vi "swerve-drive-pose-est-test.vi"(8 "error in (no error)":errorcluster) -> (0 "error out":errorcluster, 3 "Test Passed":bool)   [LabVIEW 2019]
uses:
  <vilib>/Rock Robotics/WPI/ThirdParty/JAS_Junk/TrajLib/MatBuilder_Create.vi
  <vilib>/Rock Robotics/WPI/ThirdParty/JAS_Junk/TrajLib/MatrixHelper_CoerceSize.vi
  <vilib>/Rock Robotics/WPI/ThirdParty/JAS_Junk/TrajLib/Util_CalcDist.vi
  <vilib>/Analysis/1siggen.llb/Gaussian White Noise.vi
  <vilib>/Rock Robotics/WPI/ThirdParty/JAS_Junk/TrajLib/Trajectory_Library.lvlib
panel:
  out "BenchProcessing Timer Per Pass":dbl
  out "BenchTotalTime":dbl
  out "BenchTotalPasses":dbl
  out "MaxErrPassed":bool
  out "TotalPassed":bool
  out "EerrSumNormalized":dbl
  out "Error Sum":dbl
  out "Max Error":dbl
  out "Using Vision":bool
  in  "UseVIsion":bool=TRUE
  out "VIsionUpdates":i32
  out "TotalTImeSecs":dbl
  out "Position Graph":cluster{dbl[], dbl[]}[](graph)
  out "PoesEstCreateErr":bool
  # "< 0.42"
  # "< 0.25"
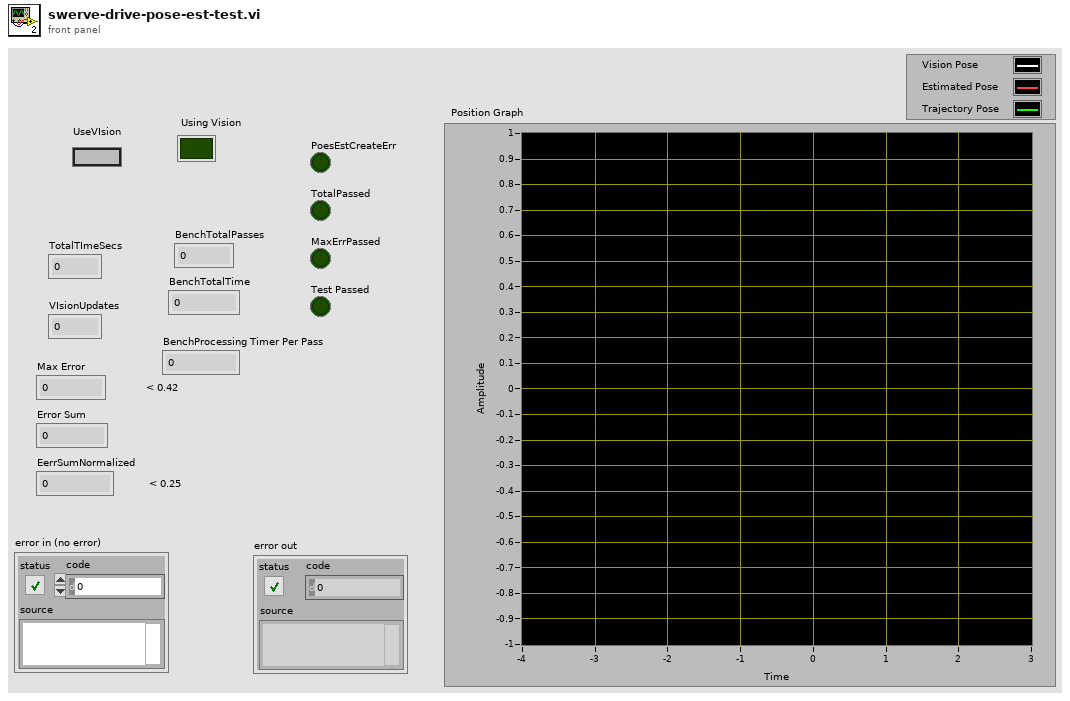
[diagram p1: front panel]
types:
  T1 = typedef "Trajectory_Library.lvlib/TRANSLATION2D.ctl" = cluster{"X":dbl, "Y":dbl}
  T2 = typedef "Trajectory_Library.lvlib/ROTATION2D.ctl" = cluster{"VALUE":dbl, "COS":dbl, "SIN":dbl}
  T3 = typedef "Trajectory_Library.lvlib/POSE2D.ctl" = cluster{"TRANSLATION":T1, "ROTATION":T2}
  T4 = typedef "NI_Matrix.lvlib/RealMatrix.ctl" = dbl[][]
  T5 = typedef "Trajectory_Library.lvlib/SWERVE_DRIVE_KINEMATICS.ctl" = cluster{"NumModules":i32, "InverseKinematics":T4, "ForwardKinematics":T4, "Modules":T1[], "PrevCoR":T1}
  T6 = typedef "Trajectory_Library.lvlib/TRAJ_CONFIG.ctl" = cluster{"MaxVelocity":dbl, "Max Acceleration":dbl, "StartVelocity":dbl, "End Velocity":dbl, "Reversed":bool, "DiffDrKineConstntDefined":bool, "CentAcellConstntDefined":bool, "DiffDrVoltConstntDefined":bool, "DIFF_DRIVE_KINE_CONSTRAINT":T7, "CENTRIPETAL_ACCEL_CONSTRAINT":T9, "SwerveDrKineConstntDefined":bool, "SWERVE_DRIVE_KINE_CONSTRAINT":T10, "DIFF_DRIVE_VOLTAGE_CONSTRAINT":T11, "MECANUM_DRIVE_KINE_CONSTRAINT":T13, "MecanumDrKineConstntDefined":bool}
  T7 = typedef "Trajectory_Library.lvlib/TRAJ_CONSTRAINT_DIIF_DRIVE_KINEMATICS.ctl" = cluster{"Max Speed (M/S)":dbl, "DIFF_DRIVE_KINEMATICS":T8, "Max Accel (M/S2)":dbl}
  T8 = typedef "Trajectory_Library.lvlib/DIFF_DRIVE_KINEMATICS.ctl" = cluster{"TrackWidth_Meters":dbl}
  T9 = typedef "Trajectory_Library.lvlib/TRAJ_CONSTRAINT_CENTRIPETAL_ACCEL.ctl" = cluster{"Max Cent Accel":dbl}
  T10 = typedef "Trajectory_Library.lvlib/TRAJ_CONSTRAINT_SWERVE_DRIVE_KINEMATICS.ctl" = cluster{"Max Speed (M/S)":dbl, "SwerveKinematics":T5}
  T11 = typedef "Trajectory_Library.lvlib/TRAJ_CONSTRAINT_DIIF_DRIVE_VOLTAGE.ctl" = cluster{"Max Voltage":dbl, "DIFF_DRIVE_KINEMATICS":T8, "SIMPLE_MOTOR_FF":T12}
  T12 = typedef "Trajectory_Library.lvlib/SIMPLE_MOTOR_FF.ctl" = cluster{"Ks":dbl, "Kv":dbl, "Ka":dbl}
  T13 = typedef "Trajectory_Library.lvlib/TRAJ_CONSTRAINT_MECA_DRIVE_KINEMATICS.ctl" = cluster{"Max Speed (M/S)":dbl, "MECA_DRIVE_KINEMATICS":T14}
  T14 = typedef "Trajectory_Library.lvlib/MECA_DRIVE_KINEMATICS.ctl" = cluster{"FrontLeft":T1, "FrontRight":T1, "RearLeft":T1, "RearRight":T1, "InverseKinematics":T4, "ForwardKinematics":T4, "PrevCoR":T1}
  T15 = typedef "Trajectory_Library.lvlib/SWERVE_DRIVE_POSE_EST.ctl" = cluster{"M_VisionContR":T4, "m_nominal_dT":dbl, "m_PrevTime_Sec":dbl, "m_GyroOffset":T2, "m_PrevAngle":T2, "m_Observer":T16, "m_latencyCompensator":T19, "m_kinematics":T5}
  T16 = typedef "Trajectory_Library.lvlib/UNSCENTED_KALMAN_FILTER.ctl" = cluster{"m_P":T4, "m_xHat":T4, "States":i32, "Outputs":i32, "m_ContR":T4, "m_ContQ":T4, "m_SigmasF":T4, "m_dT_Sec":dbl, "MERWE_SCALED_SIGMA_PTS":T17, "meanFuncX":T18, "meanFuncY":T18, "residualFuncX":T18, "residualFuncY":T18, "addFuncX":T18, "addFuncXExtra":variant, "residualFuncYExtra":variant, "residualFuncXExtra":variant, "MeanFuncYExtra":variant, "MeanFuncXExtra":variant, "Inputs":i32}
  T17 = typedef "Trajectory_Library.lvlib/MERWE_SCALED_SIGMA_PTS.ctl" = cluster{"m_Wm":T4, "States":i32, "Alpha":dbl, "m_Wc":T4, "Kappa":i32}
  T18 = typedef "Trajectory_Library.lvlib/CALLBACK_FUNC_TYPE.ctl" = refnum<vi>
  T19 = typedef "Trajectory_Library.lvlib/KALMAN_FILTER_LATENCY_COMP.ctl" = cluster{"m_pastObserverSnapshots ":T20[]}
  T20 = typedef "Trajectory_Library.lvlib/OBSERVER_SNAP_LIST_ITEM.ctl" = cluster{"TimeStamp":dbl, "OBSERVER_SNAPSHOT":T21}
  T21 = typedef "Trajectory_Library.lvlib/OBSERVER_SNAPSHOT.ctl" = cluster{"ErrorCoVariance":T4, "xHat":T4, "LocalMeasurements":T4, "Inputs":T4}
  T22 = typedef "Trajectory_Library.lvlib/TRAJECTORY.ctl" = cluster{"TotalTImeSecs":dbl, "States":T23[]}
  T23 = typedef "Trajectory_Library.lvlib/TRAJ_STATE.ctl" = cluster{"TimeSeconds":dbl, "Velocity":dbl, "Acceleration":dbl, "POSE":T3, "Curvature":dbl}
  T24 = typedef "Trajectory_Library.lvlib/CHASSIS_SPEEDS.ctl" = cluster{"vX":dbl, "vY":dbl, "vOmega":dbl}
  T25 = typedef "Trajectory_Library.lvlib/SWERVE_DRIVE_MODULE_STATE.ctl" = cluster{"Speed":dbl, "Angle":T2}
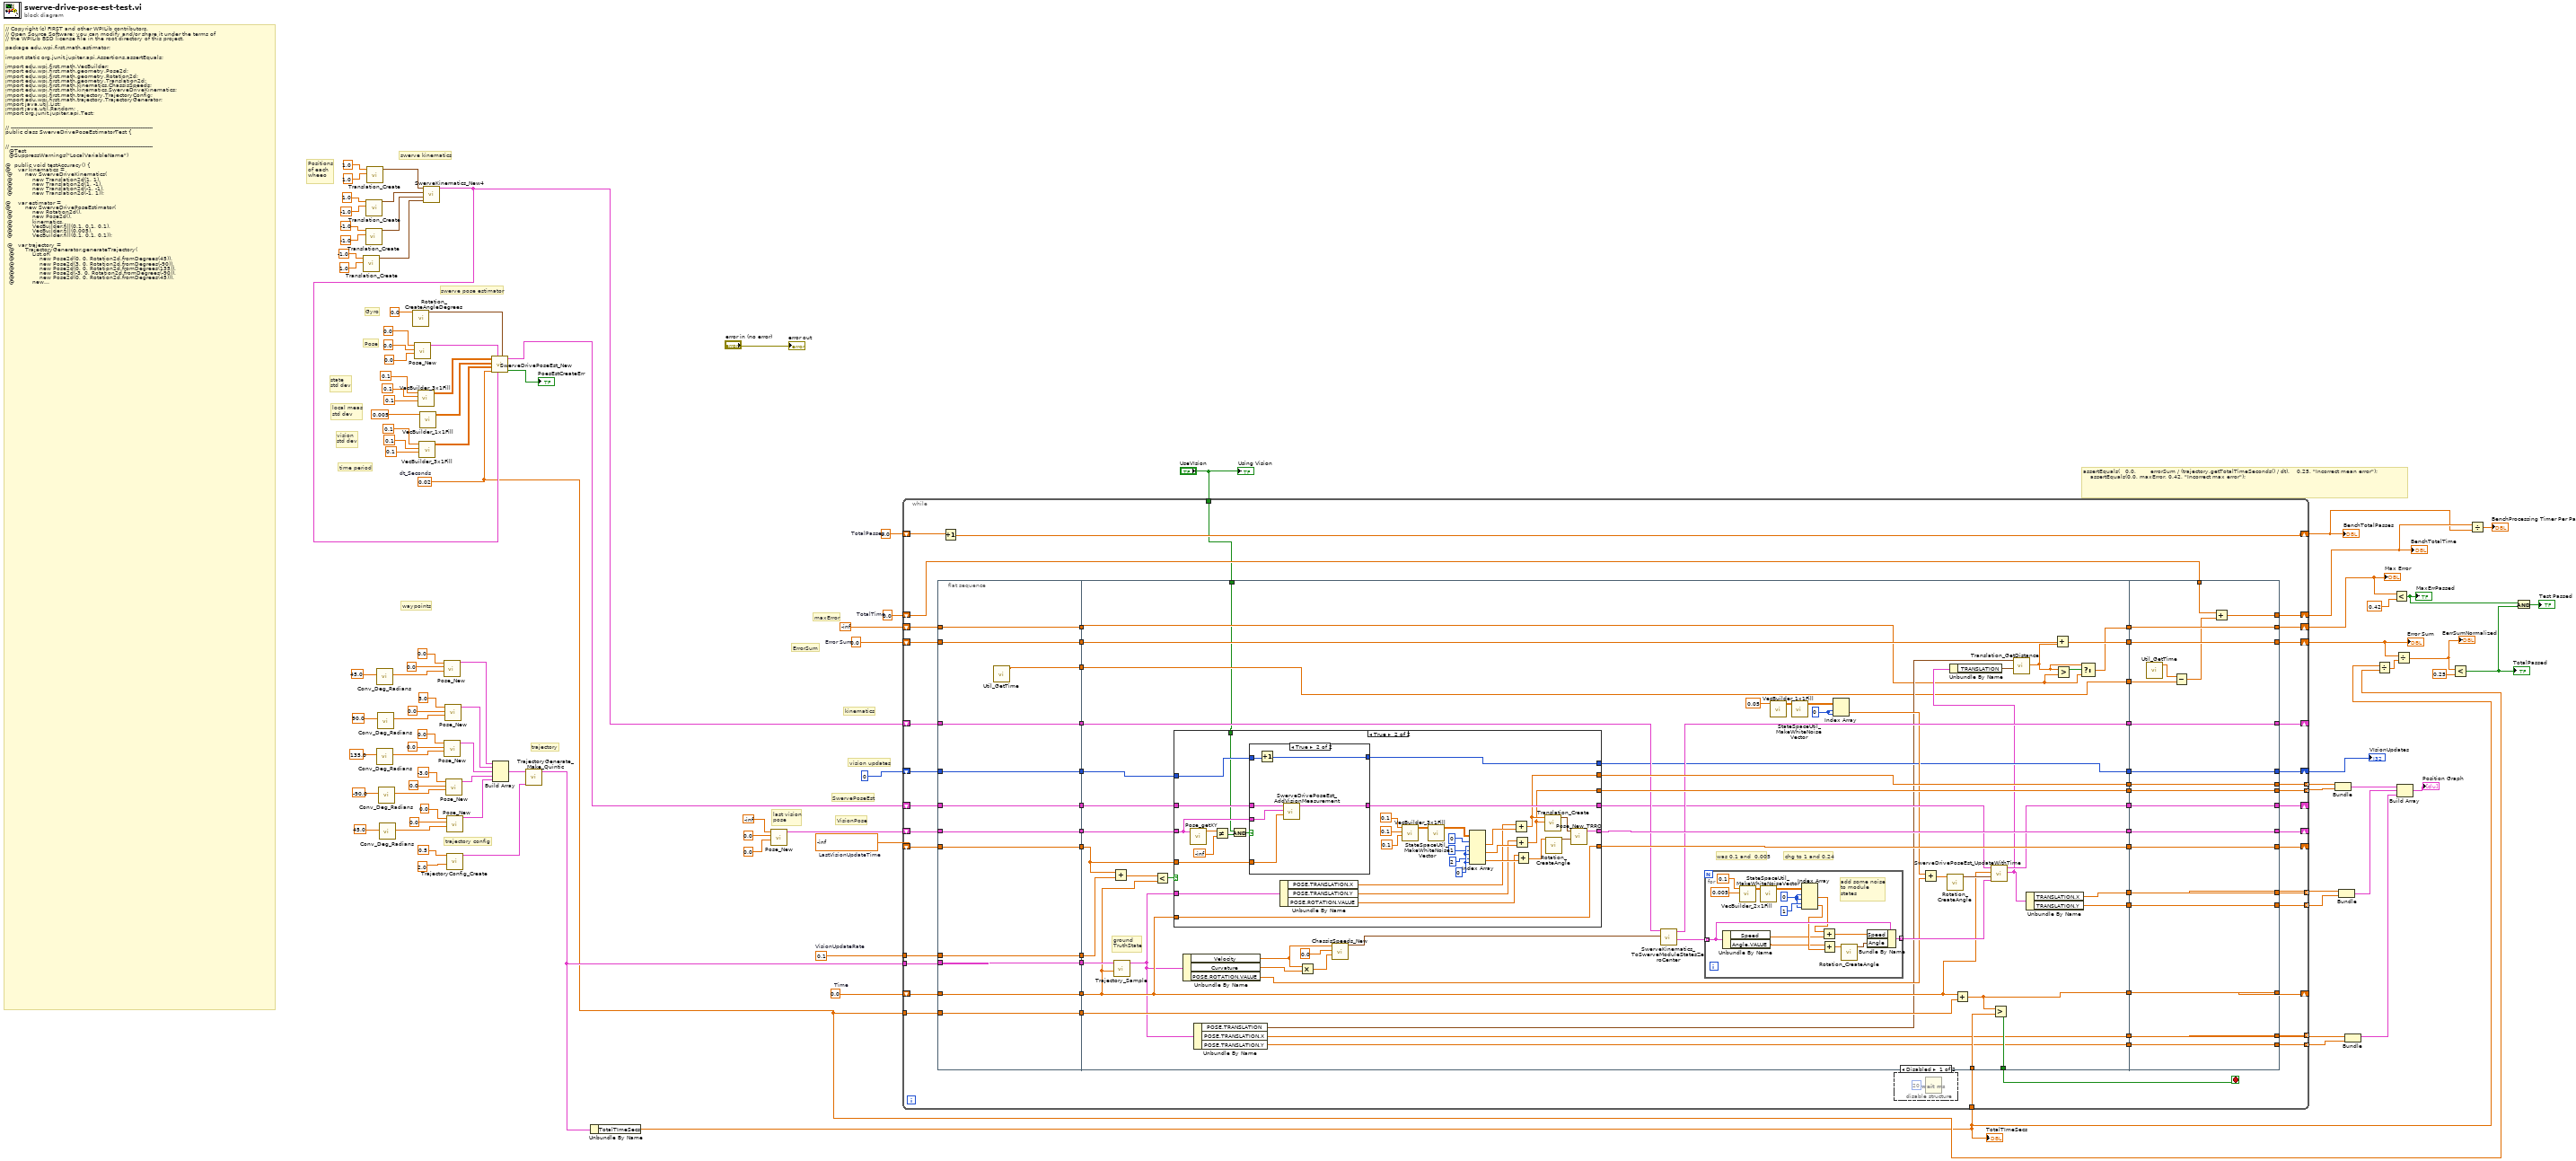
[diagram p0: block diagram]
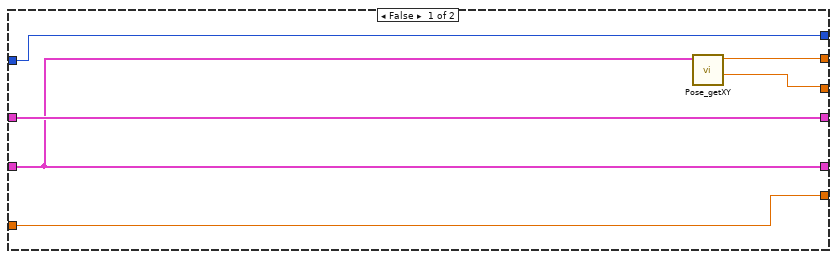
[diagram p3: hidden frame]
diagram:
  w6 = 0.0  # TotalPasses
  w7 = 0.0  # TotalTime
  w19 = 0.0  # Error Sum
  w39 = 0.1  # VisionUpdateRate
  w40 = -inf  # LastVisionUpdateTime
  w42 = 0.0  # Time
  w17 = 0.02  # dt_Seconds
  # "assertEquals(   0.0,        errorSum / (trajectory.getTotalTimeSeconds() / dt),    0.25, \"Incorrect mean error\");\n    assertEquals(0.0, maxError, 0.42, \"Incorrect max error\");"
  # "ErrorSum"
  # "maxError"
  # "vision updates"
  # "kinematics"
  # "SwervePoseEst"
  # "VisionPose"
  # "last vision\npose"
  # "time period"
  # "vision \nstd dev"
  # "local meas\nstd dev"
  # "state\nstd dev"
  # "Pose"
  # "Gyro"
  # "Positions\nof each\nwheeo"
  # "swerve pose estimator"
  # "swerve kinematics"
  # "trajectory config"
  # "trajectory"
  # "waypoints"
  # "// Copyright (c) FIRST and other WPILib contributors.\n// Open Source Software; you can modify and/or share it under the terms of\n// the WPILib BSD license file in the root directory of this project.\n\npackage edu.wpi.first.math.estimator;\n\nimport static org.junit.jupiter.api.Assertions.assertEquals;\n\nimport edu.wpi.first.math.VecBuilder;\nimport edu.wpi.first.math.geometry.Pose2d;\nimport edu.wpi.first.math.geometry.Rotation2d;\nimport edu.wpi.first.math.geometry.Translation2d;\nimport edu.wpi.first.math.kinematics.ChassisSpeeds;\nimport edu.wpi.first.math.kinematics.SwerveDriveKinematics;\nimport edu.wpi.first.math.trajectory.TrajectoryConfig;\nimport edu.wpi.first.math.trajectory.TrajectoryGenerator;\nimport java.util.List;\nimport java.util.Random;\nimport org.junit.jupiter.api.Test;\n\n\n// -------------------------------------------------------------------------------\npublic class SwerveDrivePoseEstimatorTest {\n\n\n// -------------------------------------------------------------------------------\n  @Test\n  @SuppressWarnings(\"LocalVariableName\")\n\n@  public void testAccuracy() {\n@    var kinematics =\n @       new SwerveDriveKinematics(\n @           new Translation2d(1, 1),\n @           new Translation2d(1, -1),\n @           new Translation2d(-1, -1),\n @           new Translation2d(-1, 1));\n\n@    var estimator =\n@        new SwerveDrivePoseEstimator(\n @           new Rotation2d(),\n @           new Pose2d(),\n @           kinematics,\n @           VecBuilder.fill(0.1, 0.1, 0.1),\n @           VecBuilder.fill(0.005),\n @           VecBuilder.fill(0.1, 0.1, 0.1));\n\n @   var trajectory =\n  @      TrajectoryGenerator.generateTrajectory(\n  @          List.of(\n  @              new Pose2d(0, 0, Rotation2d.fromDegrees(45)),\n  @              new Pose2d(3, 0, Rotation2d.fromDegrees(-90)),\n  @              new Pose2d(0, 0, Rotation2d.fromDegrees(135)),\n  @              new Pose2d(-3, 0, Rotation2d.fromDegrees(-90)),\n  @              new Pose2d(0, 0, Rotation2d.fromDegrees(45))),\n  @          new TrajectoryConfig(0.5, 2));\n\n    var rand = new Random(4915);\n\n@    final double dt = 0.02;\n @   double t = 0.0;\n\n @   final double visionUpdateRate = 0.1;\n  @  Pose2d lastVisionPose = null;\n @   double lastVisionUpdateTime = Double.NEGATIVE_INFINITY;\n\n @   double maxError = Double.NEGATIVE_INFINITY;\n  @  double errorSum = 0;\n\n@    while (t <= trajectory.getTotalTimeSeconds()) {\n\n @     var groundTruthState = trajectory.sample(t);\n\n @     if (lastVisionUpdateTime + visionUpdateRate < t) {\n  @      if (lastVisionPose != null) {\n   @       estimator.addVisionMeasurement(lastVisionPose, lastVisionUpdateTime);\n   @     }\n\n @       lastVisionPose =\n @           new Pose2d(\n @               new Translation2d(\n  @                  groundTruthState.poseMeters.getTranslation().getX() + rand.nextGaussian() * 0.1,\n  @                  groundTruthState.poseMeters.getTranslation().getY()\n  @                      + rand.nextGaussian() * 0.1),\n @               new Rotation2d(rand.nextGaussian() * 0.1)\n  @                  .plus(groundTruthState.poseMeters.getRotation()));\n\n  @      lastVisionUpdateTime = t;\n  @    }  // end if \n\n  @    var moduleStates =\n   @       kinematics.toSwerveModuleStates(\n    @          new ChassisSpeeds(\n     @             groundTruthState.velocityMetersPerSecond,\n      @            0.0,\n     @             groundTruthState.velocityMetersPerSecond\n    @                  * groundTruthState.curvatureRadPerMeter));\n\n @     for (var moduleState : moduleStates) {\n  @      moduleState.angle = moduleState.angle.plus(new Rotation2d(rand.nextGaussian() * 0.005));\n @       moduleState.speedMetersPerSecond += rand.nextGaussian() * 0.1;\n @     }\n\n\n @     var xHat =\n  @        estimator.updateWithTime(\n  @            t,\n  @            groundTruthState.poseMeters.getRotation()\n  @                .plus(new Rotation2d(rand.nextGaussian() * 0.05)),\n  @            moduleStates);\n\n @     double error =\n @         groundTruthState.poseMeters.getTranslation().getDistance(xHat.getTranslation());\n @     if (error > maxError) {\n  @      maxError = error;\n  @    }\n  @    errorSum += error;\n\n@      t += dt;\n @   }    // END OF LOOP\n\n    assertEquals(\n        0.0, errorSum / (trajectory.getTotalTimeSeconds() / dt), 0.25, \"Incorrect mean error\");\n    assertEquals(0.0, maxError, 0.42, \"Incorrect max error\");\n  }\n}"
  n1 = call <vilib>:"Translation_Create.vi"("Y"=1.0, "X"=-1.0) -> ("TRANSLATION"=w60:T1)  [unwired: 9 in]
  n2 = call <vilib>:"Translation_Create.vi"("Y"=-1.0, "X"=-1.0) -> ("TRANSLATION"=w61:T1)  [unwired: 9 in]
  n3 = call <vilib>:"Translation_Create.vi"("Y"=-1.0, "X"=1.0) -> ("TRANSLATION"=w62:T1)  [unwired: 9 in]
  n4 = call <vilib>:"Translation_Create.vi"("Y"=1.0, "X"=1.0) -> ("TRANSLATION"=w63:T1)  [unwired: 9 in]
  n5 = call <vilib>:"Conv_Deg_Radians.vi"("Degress"=45.0 ("Heading")) -> ("Radians"=w77:dbl)  [unwired: 10 in]
  n6 = call <vilib>:"Conv_Deg_Radians.vi"("Degress"=135.0 ("Heading")) -> ("Radians"=w85:dbl)  [unwired: 10 in]
  n7 = call <vilib>:"Conv_Deg_Radians.vi"("Degress"=90.0 ("Heading")) -> ("Radians"=w81:dbl)  [unwired: 10 in]
  n8 = call <vilib>:"Conv_Deg_Radians.vi"("Degress"=-90.0 ("Heading")) -> ("Radians"=w89:dbl)  [unwired: 10 in]
  n9 = call <vilib>:"Conv_Deg_Radians.vi"("Degress"=45.0 ("Heading")) -> ("Radians"=w93:dbl)  [unwired: 10 in]
  n10 = call <vilib>:"Rotation_CreateAngleDegrees.vi"("Angle_Degrees"=0.0) -> ("ROTATION"=w59:T2)  [unwired: 10 in]
  n11 = call <vilib>:"Pose_New.vi"("Heading"=0.0, "Y"=0.0, "X"=0.0) -> ("out POSe"=w57:T3)  [unwired: 8 in]
  n12 = call <vilib>:"VecBuilder_3x1Fill.vi"("R2"=0.1 ("element"), "R1"=0.1 ("element"), "R0"=0.1 ("element")) -> ("output matrix"=w49:T4)  [unwired: 8 in]
  n13 = call <vilib>:"VecBuilder_3x1Fill.vi"("R2"=0.1 ("element"), "R1"=0.1 ("element"), "R0"=0.1 ("element")) -> ("output matrix"=w44:T4)  [unwired: 8 in]
  n14 = call <vilib>:"VecBuilder_1x1Fill.vi"("R0_C0"=0.005 ("element")) -> ("output matrix"=w48:T4)  [unwired: 10 in]
  n15 = call <vilib>:"SwerveKinematics_New4.vi"("wheel 3"=w60, "wheel 2"=w61, "wheel 1"=w62, "wheel 0"=w63) -> ("SWERVE_DRIVE_KINEMATICS"=w32:T5)  [unwired: 7 in]
  n16 = call <vilib>:"Pose_New.vi"("Heading"=w77, "Y"=0.0, "X"=0.0) -> ("out POSe"=w76:T3)  [unwired: 8 in]
  n17 = call <vilib>:"Pose_New.vi"("Heading"=w85, "Y"=0.0, "X"=0.0) -> ("out POSe"=w73:T3)  [unwired: 8 in]
  n18 = call <vilib>:"Pose_New.vi"("Heading"=w81, "Y"=0.0, "X"=3.0) -> ("out POSe"=w74:T3)  [unwired: 8 in]
  n19 = call <vilib>:"Pose_New.vi"("Heading"=w89, "Y"=0.0, "X"=-3.0) -> ("out POSe"=w72:T3)  [unwired: 8 in]
  n20 = call <vilib>:"Pose_New.vi"("Heading"=w93, "Y"=0.0, "X"=0.0) -> ("out POSe"=w98:T3)  [unwired: 8 in]
  n21 = call <vilib>:"TrajectoryConfig_Create.vi"("MaxAcceleration"=2.0, "MaxVelocity"=0.5) -> ("TRAJECTORY_CONFIG"=w95:T6)  [unwired: 9 in]
  n22 = call <vilib>:"SwerveDrivePoseEst_New.vi"("gyroAngle"=w59, "SwerveKinematics"=w32, "InitialPose"=w57, "dt_Seconds"=w17, "VisionMeasurementStdDevs"=w44, "LocalMeasurementStdDevs"=w48, "StateStdDevs"=w49) -> ("Error"=→"PoesEstCreateErr":bool, "SwerveDrivePoseEstimate"=w34:T15)  [unwired: 3 in]
  n23 = Build Array(w76, w74, w73, w72, w98) -> (w96:T3[])
  n24 = call <vilib>:"TrajectoryGenerate_Make_Quintic.vi"("traj_config"=w95, "waypointPOSE"=w96) -> ("TRAJECTORY"=w41:T22)  [unwired: 8 in, 1 out]
  n25 = Unbundle By Name(w41) -> ("TotalTImeSecs"=w10:dbl)
  "TotalTImeSecs" <- w10
  n26 = call <vilib>:"Pose_New.vi"("Heading"=0.0, "Y"=0.0, "X"=-inf) -> ("out POSe"=w35:T3)  [unwired: 8 in]
  n27 = while {
    tunnel: w17 -> [w159]
    shift-right: [w158] -> _
    shift-left: w42 -> [w145]
    tunnel: w41 -> [w156]
    tunnel: w10 -> [w157]
    shift-right: [w150] -> _
    shift-left: w40 -> [w152]
    tunnel: w39 -> [w155]
    shift-right: [w151] -> _
    shift-left: w35 -> [w154]
    shift-right: [w144] -> _
    shift-left: w34 -> [w153]
    tunnel: [w149] -> w33 mode=indexing
    tunnel: [w148] -> w31 mode=indexing
    shift-right: [w146] -> _
    shift-left: w32 -> [w147]
    tunnel: [w143] -> w30 mode=indexing
    tunnel: [w142] -> w29 mode=indexing
    shift-right: [w140] -> w24
    shift-left: 0 -> [w141]
    tunnel: [w139] -> w23 mode=indexing
    tunnel: [w138] -> w22 mode=indexing
    shift-right: [w135] -> w15
    shift-left: -inf -> [w134]
    shift-right: [w136] -> w18
    shift-left: w19 -> [w137]
    shift-right: [w105] -> w5
    shift-left: w7 -> [w104]
    shift-right: [w102] -> w4
    shift-left: w6 -> [w103]
    tunnel: "UseVIsion" -> [w101]
    stop <- w133 stop-if-true
    n28 = flat-sequence {
      tunnel: w134 -> [w162]
      tunnel: w137 -> [w163]
      tunnel: w141 -> [w164]
      tunnel: w145 -> [w165]
      tunnel: w147 -> [w166]
      tunnel: w152 -> [w167]
      tunnel: w153 -> [w168]
      tunnel: w154 -> [w169]
      tunnel: w155 -> [w170]
      tunnel: w156 -> [w171]
      tunnel: w159 -> [w172]
      tunnel: [w172] -> w132
      tunnel: [w171] -> w131
      tunnel: [w170] -> w130
      tunnel: [w169] -> w129
      tunnel: [w168] -> w128
      tunnel: [w167] -> w127
      tunnel: [w166] -> w126
      tunnel: [w165] -> w125
      tunnel: [w164] -> w124
      tunnel: [w163] -> w123
      tunnel: [w162] -> w122
      tunnel: [w161] -> w107
      tunnel: [w224] -> w133
      tunnel: w157 -> [w222]
      tunnel: w132 -> [w225]
      tunnel: w131 -> [w221]
      tunnel: w130 -> [w219]
      tunnel: w129 -> [w217]
      tunnel: w128 -> [w216]
      tunnel: w127 -> [w215]
      tunnel: w126 -> [w205]
      tunnel: w125 -> [w192]
      tunnel: w124 -> [w188]
      tunnel: w123 -> [w180]
      tunnel: w122 -> [w175]
      tunnel: [w223] -> w121
      tunnel: [w214] -> w120
      tunnel: [w213] -> w119
      tunnel: [w212] -> w118
      tunnel: [w211] -> w117
      tunnel: [w204] -> w116
      tunnel: [w191] -> w115
      tunnel: [w190] -> w114
      tunnel: [w189] -> w113
      tunnel: [w187] -> w112
      tunnel: [w185] -> w111
      tunnel: [w184] -> w110
      tunnel: [w179] -> w109
      tunnel: [w176] -> w108
      tunnel: w107 -> [w174]
      tunnel: [w174] -> w106
      tunnel: w101 -> [w173]
      tunnel: [w294] -> w135
      tunnel: [w295] -> w136
      tunnel: [w296] -> w138
      tunnel: [w297] -> w139
      tunnel: [w298] -> w140
      tunnel: [w299] -> w142
      tunnel: [w300] -> w143
      tunnel: [w301] -> w144
      tunnel: [w302] -> w146
      tunnel: [w303] -> w148
      tunnel: [w304] -> w149
      tunnel: [w305] -> w150
      tunnel: [w306] -> w151
      tunnel: [w307] -> w158
      tunnel: w121 -> [w307]
      tunnel: w120 -> [w306]
      tunnel: w119 -> [w305]
      tunnel: w118 -> [w304]
      tunnel: w117 -> [w303]
      tunnel: w116 -> [w302]
      tunnel: w115 -> [w301]
      tunnel: w114 -> [w300]
      tunnel: w113 -> [w299]
      tunnel: w112 -> [w298]
      tunnel: w111 -> [w297]
      tunnel: w110 -> [w296]
      tunnel: w109 -> [w295]
      tunnel: w108 -> [w294]
      tunnel: w106 -> [w292]
      tunnel: [w291] -> w105
      tunnel: w104 -> [w289]
      frame #0 {
        n29 = call <vilib>:"Util_GetTime.vi"() -> ("FPGA_Time_Seconds"=w161:dbl)  [unwired: 10 in, 1 out]
      }
      frame #1 {
        w197 = 0 ("index (col)")
        # "chg to 1 and 0.24"
        # "was 0.1 and  0.005"
        # "ground\nTruthState"
        n30 = Add(x=w215, y=w219) -> (x+y=w218:dbl)
        n31 = call <vilib>:"Trajectory_Sample.vi"("Time"=w192, "InputTRAJECTORY"=w221) -> ("OutputTRAJ_STATE"=w186:T23)  [unwired: 9 in]
        n32 = Less?(x=w218, y=w192) -> (x < y?=w220:bool)
        n33 = case shown="True" w220 {
          tunnel: w217 -> [w244 w277]
          tunnel: w216 -> [w246 w278]
          tunnel: [w246 w276] -> w202
          tunnel: w215 -> [w245 w275]
          tunnel: w186 -> [_ w268]
          tunnel: [w244 w274] -> w214
          tunnel: w192 -> [_ w254]
          tunnel: [w245 w254] -> w213
          tunnel: [w243 w253] -> w212
          tunnel: [w242 w252] -> w211
          tunnel: w188 -> [w241 w251]
          tunnel: [w241 w250] -> w187
          tunnel: w173 -> [_ w247]
          frame False {
            n34 = call <vilib>:"Pose_getXY.vi"("in POSE"=w244) -> ("Y"=w242:dbl, "X"=w243:dbl)  [unwired: 9 in]
          }
          frame True {
            w265 = 0 ("index (col)")
            n35 = call <vilib>:"Pose_getXY.vi"("in POSE"=w277) -> ("X"=w280:dbl)  [unwired: 9 in, 1 out]
            n36 = Not Equal?(x=w280, y=-inf) -> (x != y?=w248:bool)
            n37 = And(x=w247, y=w248) -> (x .and. y?=w249:bool)
            n38 = case shown="True" w249 {
              tunnel: w278 -> [w282 w288]
              tunnel: w277 -> [_ w287]
              tunnel: [w282 w286] -> w276
              tunnel: w275 -> [_ w285]
              tunnel: w251 -> [w281 w284]
              tunnel: [w281 w283] -> w250
              frame False {
              }
              frame True {
                n39 = Increment(x=w284) -> (x+1=w283:i32)
                n40 = call <vilib>:"SwerveDrivePoseEst_AddVisionMeasurement.vi"("TImeStamp_Seconds"=w285, "visionRobotPose"=w287, "in SwerveDrivePoseEstimate"=w288) -> ("OutSwerveDrivePoseEstimate"=w286:T15)  [unwired: 7 in, 1 out]
              }
            }
            n41 = Unbundle By Name(w268) -> ("POSE.TRANSLATION.X"=w257:dbl, "POSE.TRANSLATION.Y"=w256:dbl, "POSE.ROTATION.VALUE"=w255:dbl)
            n42 = call <vilib>:"VecBuilder_3x1Fill.vi"("R2"=0.1, "R1"=0.1, "R0"=0.1) -> ("output matrix"=w272:T4)  [unwired: 8 in]
            n43 = call <vilib>:"StateSpaceUtil_MakeWhiteNoiseVector.vi"("StdDevs"=w272) -> ("WhiteNoise"=w266:T4)  [unwired: 9 in, 1 out]
            n44 = Index Array(array=w266, index (row) #1=0 ("index (col)"), index (col) #1=w265, index (row) #2=1 ("index (col)"), index (col) #2=w265, index (row) #3=2 ("index (col)"), index (col) #3=w265) -> (element #1=w259:dbl, element #2=w260:dbl, element #3=w261:dbl)
            n45 = Add(x=w257, y=w259) -> (x+y=w253:dbl)
            n46 = Add(x=w256, y=w260) -> (x+y=w252:dbl)
            n47 = Add(x=w255, y=w261) -> (x+y=w258:dbl)
            n48 = call <vilib>:"Translation_Create.vi"("Y"=w252, "X"=w253) -> ("TRANSLATION"=w273:T1)  [unwired: 9 in]
            n49 = call <vilib>:"Rotation_CreateAngle.vi"("Angle"=w258) -> ("ROTATION"=w267:T2)  [unwired: 10 in]
            n50 = call <vilib>:"Pose_New_TRRO.vi"("ROTATION"=w267, "TRANSLATION"=w273) -> ("outPOSE"=w274:T3)  [unwired: 9 in]
          }
        }
        n51 = Unbundle By Name(w186) -> ("Velocity"=w208:dbl, "Curvature"=w209:dbl, "POSE.ROTATION.VALUE"=w196:dbl)
        n52 = Unbundle By Name(w186) -> ("POSE.TRANSLATION"=w183:T1, "POSE.TRANSLATION.X"=w184:dbl, "POSE.TRANSLATION.Y"=w185:dbl)
        n53 = Multiply(x=w208, y=w209) -> (x*y=w207:dbl)
        n54 = call <vilib>:"ChassisSpeeds_New.vi"("vAngular"=w207, "vY"=0.0, "vX"=w208) -> ("CHASSIS"=w206:T24)  [unwired: 8 in]
        n55 = call <vilib>:"SwerveKinematics_ToSwerveModuleStatesZeroCenter.vi"("ChassisSpeeds"=w206, "in SWERVE_DRIVE_KINEMATICS"=w205) -> ("ModuleStates"=w203:T25[], "out SWERVE_DRIVE_KINEMATICS"=w204:T5)  [unwired: 8 in]
        n56 = for {
          tunnel: w203 -> [w234] mode=indexing
          tunnel: [w226] -> w201 mode=indexing
          w235 = 0 ("index (col)")
          # "add some noise\nto module\nstates"
          n57 = Unbundle By Name(w234) -> ("Speed"=w228:dbl, "Angle.VALUE"=w227:dbl)
          n58 = call <vilib>:"VecBuilder_2x1Fill.vi"("R1"=0.005, "R0"=0.1) -> ("output matrix"=w240:T4)  [unwired: 9 in]
          n59 = call <vilib>:"StateSpaceUtil_MakeWhiteNoiseVector.vi"("StdDevs"=w240) -> ("WhiteNoise"=w237:T4)  [unwired: 9 in, 1 out]
          n60 = Index Array(array=w237, index (row) #1=w235, index (col) #1=w235, index (row) #2=1 ("index (col)"), index (col) #2=w235) -> (element #1=w229:dbl, element #2=w230:dbl)
          n61 = Add(x=w229, y=w228) -> (x+y=w231:dbl)
          n62 = Add(x=w227, y=w230) -> (x+y=w232:dbl)
          n63 = call <vilib>:"Rotation_CreateAngle.vi"("Angle"=w232) -> ("ROTATION"=w233:T2)  [unwired: 10 in]
          n64 = Bundle By Name(cluster=w234, "Speed"=w231, "Angle"=w233) -> (w226:T25)
        }
        n65 = call <vilib>:"VecBuilder_1x1Fill.vi"("R0_C0"=0.05 ("R0")) -> ("output matrix"=w200:T4)  [unwired: 10 in]
        n66 = call <vilib>:"StateSpaceUtil_MakeWhiteNoiseVector.vi"("StdDevs"=w200) -> ("WhiteNoise"=w198:T4)  [unwired: 9 in, 1 out]
        n67 = Index Array(array=w198, index (row)=w197, index (col)=w197) -> (element=w195:dbl)
        n68 = Add(x=w195, y=w196) -> (x+y=w194:dbl)
        n69 = call <vilib>:"Rotation_CreateAngle.vi"("Angle"=w194) -> ("ROTATION"=w193:T2)  [unwired: 10 in]
        n70 = Add(x=w192, y=w225) -> (x+y=w223:dbl)
        n71 = call <vilib>:"SwerveDrivePoseEst_UpdateWithTime.vi"("SweveModuleStates"=w201, "GyroAngle"=w193, "CurrentTimeSeconds"=w192, "in SwerveDrivePoseEstimate"=w202) -> ("Estimated Pose"=w182:T3, "Out SwerveDrivePoseEstimate"=w191:T15)  [unwired: 5 in, 1 out]
        n72 = Unbundle By Name(w182) -> ("TRANSLATION"=w181:T1)
        n73 = Greater?(x=w223, y=w222) -> (0:w224:bool)
        n74 = call <vilib>:"Translation_GetDistance.vi"("other Translation"=w181, "In Translation"=w183) -> ("Distance"=w177:dbl)  [unwired: 9 in]
        n75 = Unbundle By Name(w182) -> ("TRANSLATION.X"=w190:dbl, "TRANSLATION.Y"=w189:dbl)
        n76 = Add(x=w180, y=w177) -> (x+y=w179:dbl)
        n77 = Greater?(x=w177, y=w175) -> (0:w178:bool)
        n78 = Select(t=w177, s=w178, f=w175) -> (s? t:f=w176:dbl)
      }
      frame #2 {
        n79 = call <vilib>:"Util_GetTime.vi"() -> ("FPGA_Time_Seconds"=w293:dbl)  [unwired: 10 in, 1 out]
        n80 = Subtract(x=w293, y=w292) -> (x-y=w290:dbl)
        n81 = Add(x=w289, y=w290) -> (x+y=w291:dbl)
      }
    }
    n82 = Increment(x=w103) -> (x+1=w102:dbl)
    n83 = disable-structure shown="Disabled" {
      frame Disabled {
        n84 = Wait (ms)(milliseconds to wait=u32 20) -> ()  [unwired: 1 out]
      }
      frame Enabled {
      }
    }
  }
  "VIsionUpdates" <- w24
  "Max Error" <- w15
  "Error Sum" <- w18
  "BenchTotalPasses" <- w4
  "BenchTotalTime" <- w5
  n85 = Bundle(w33, w31) -> (w28:cluster{dbl[], dbl[]})  [unwired: 1 in]
  n86 = Bundle(w30, w29) -> (w27:cluster{dbl[], dbl[]})  [unwired: 1 in]
  n87 = Bundle(w22, w23) -> (w21:cluster{dbl[], dbl[]})  [unwired: 1 in]
  n88 = Divide(x=w10, y=w17) -> (x/y=w8:dbl)
  n89 = Less?(x=w15, y=0.42) -> (x < y?=w13:bool)
  "MaxErrPassed" <- w13
  n90 = Divide(x=w18, y=w8) -> (x/y=w9:dbl)
  "EerrSumNormalized" <- w9
  n91 = Build Array(w28, w27, w21) -> (→"Position Graph":cluster{dbl[], dbl[]}[])
  n92 = Less?(x=w9, y=0.25) -> (x < y?=w12:bool)
  "TotalPassed" <- w12
  n93 = Divide(x=w5, y=w4) -> (x/y=→"BenchProcessing Timer Per Pass":dbl)
  n94 = And(x=w13, y=w12) -> (x .and. y?=→"Test Passed":bool)
  "Using Vision" <- "UseVIsion"
  "error out" <- "error in (no error)"
